vi "HTVacuum.ReadDI.vi"(0 "i ref in":refnum<vi>, 2 "Port#":u32, 5 "error in (no error)":errorcluster) -> (14 "i ref out":refnum<vi>, 16 "Port Status":bool, 19 "error out":errorcluster)   [LabVIEW 2014, in "HTVacuum.lvlib"]
doc: "Reads the attribute data of the object after the access to the data has been locked by the \"acquire\" method. If the attribute data has been locked already, this methods waits until the attribute data is unlocked or there is a timeout.\n\nThe attribute data must be unlocked using the methods \"release\" or \"set modified data\".\n\nLicense Agreement for this software:\n\nCopyright (C)\nGesellschaft für Schwerionenforschung, GSI\nPlanckstr. 1\n64291 Darmstadt\nGermany\n\nContact: D.Beck@gsi.de \n\nThis program is free software; you can redistribute it and/or modify it under the terms of the GNU General Public License as published by the Free Software Foundation; either version 2 of the license, or (at your option) any later version.\n\nThis program is distributed in the hope that it will be useful, but WITHOUT ANY WARRANTY; without even the implied warranty of MERCHANTABILITY or FITNESS FOR A PARTICULAR PURPOSE. See the GNU General License for more details (http://www.gnu.org).\n\nGesellschaft für Schwerionenforschung, GSI\nPlanckstr. 1, 64291 Darmstadt, Germany\nFor all questions and ideas contact: M.Richter@gsi.de, H.Brand@gsi.de or D.Beck@gsi.de.\nLast update: 17-JUN-2004"
uses:
  HTVacuum.lvlib
  CSinstr.lib/M&M/_ica01/ica-Lib SubVIs/M&M SubVIs/M&M USB DIO Get Status.vi
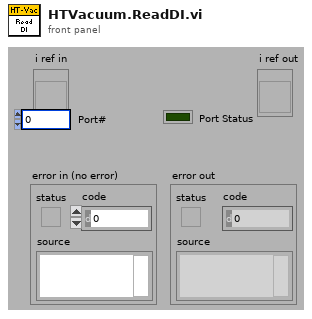
[diagram p1: front panel]
types:
  T1 = typedef "HTVacuum.lvlib/HTVacuum.i attribute.ctl" = cluster{"USB-Handle":cluster{"Write handle":i32, "Read handle":i32}}
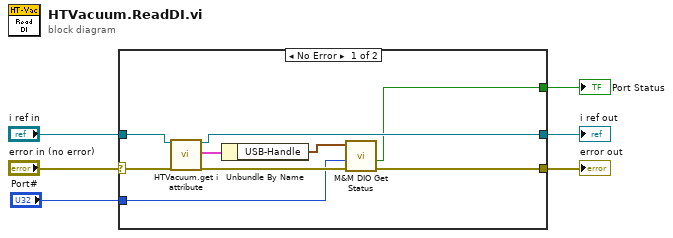
[diagram p0: block diagram]
diagram:
  n1 = case shown="No Error" "error in (no error)" {
    selector: "error in (no error)" -> [w15 w17]
    tunnel: [w9 w17] -> w5
    tunnel: "i ref in" -> [w14 w16]
    tunnel: [w13 w16] -> w3
    tunnel: "Port#" -> [w8 _]
    tunnel: [w7 _] -> w1
    frame No Error {
      n2 = call "HTVacuum.get i attribute.vi"("i ref in"=w14, "error in (no error)"=w15) -> ("i ref out"=w13:refnum<vi>, "i attribute"=w12:T1, "error out"=w10:errorcluster)  [unwired: 15 in]
      n3 = Unbundle By Name(w12) -> ("USB-Handle"=w11:cluster{"Write handle":i32, "Read handle":i32})
      n4 = call-poly "M&M DIO Get Status.vi"("error in (no error)"=w10, "Port # (1)"=w8, "USB-Handles in"=w11) -> ("error out"=w9:errorcluster, "Port Status"=w7:bool)  [unwired: 3 in, 3 out]
    }
    frame Error {
    }
  }
  "error out" <- w5
  "i ref out" <- w3
  "Port Status" <- w1
